vi "Acquire Data.vi"(8 "error in (no error)":errorcluster caption="entrée d'erreur (pas d'erreur)", 11 "Maestro Acq en entrée":refnum<class "Maestro Acq.lvclass">) -> (0 "error out":errorcluster caption="sortie d'erreur", 3 "Maestro Acq en sortie":refnum<class "Maestro Acq.lvclass">)   [LabVIEW 2021, in "Maestro Acq.lvclass"]
uses:
  Maestro Acq.lvclass
  Maestro Acq.lvclass/Maestro Acq.ctl
  4792ea48-66b7-418b-978d-52d7629da4b6.vi
panel:
  out "tableau 2":string[](array[string])
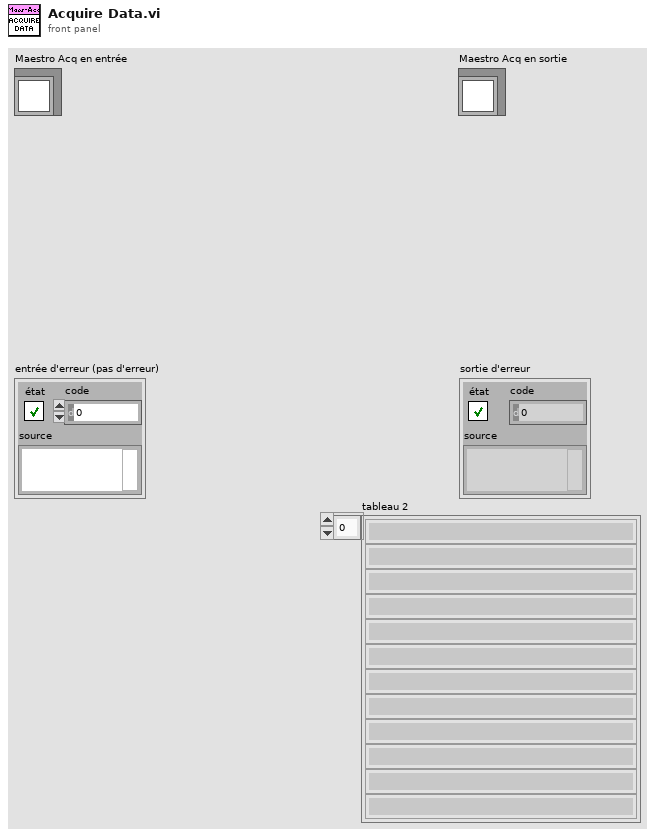
[diagram p1: front panel]
types:
  T1 = enum16{"Standard", "Buffered", "CRLF", "Immediate"}
  T2 = cluster{"Tps(s)":dbl[], "Puiss.":dbl, "Waveform":waveform(dbl)[]}
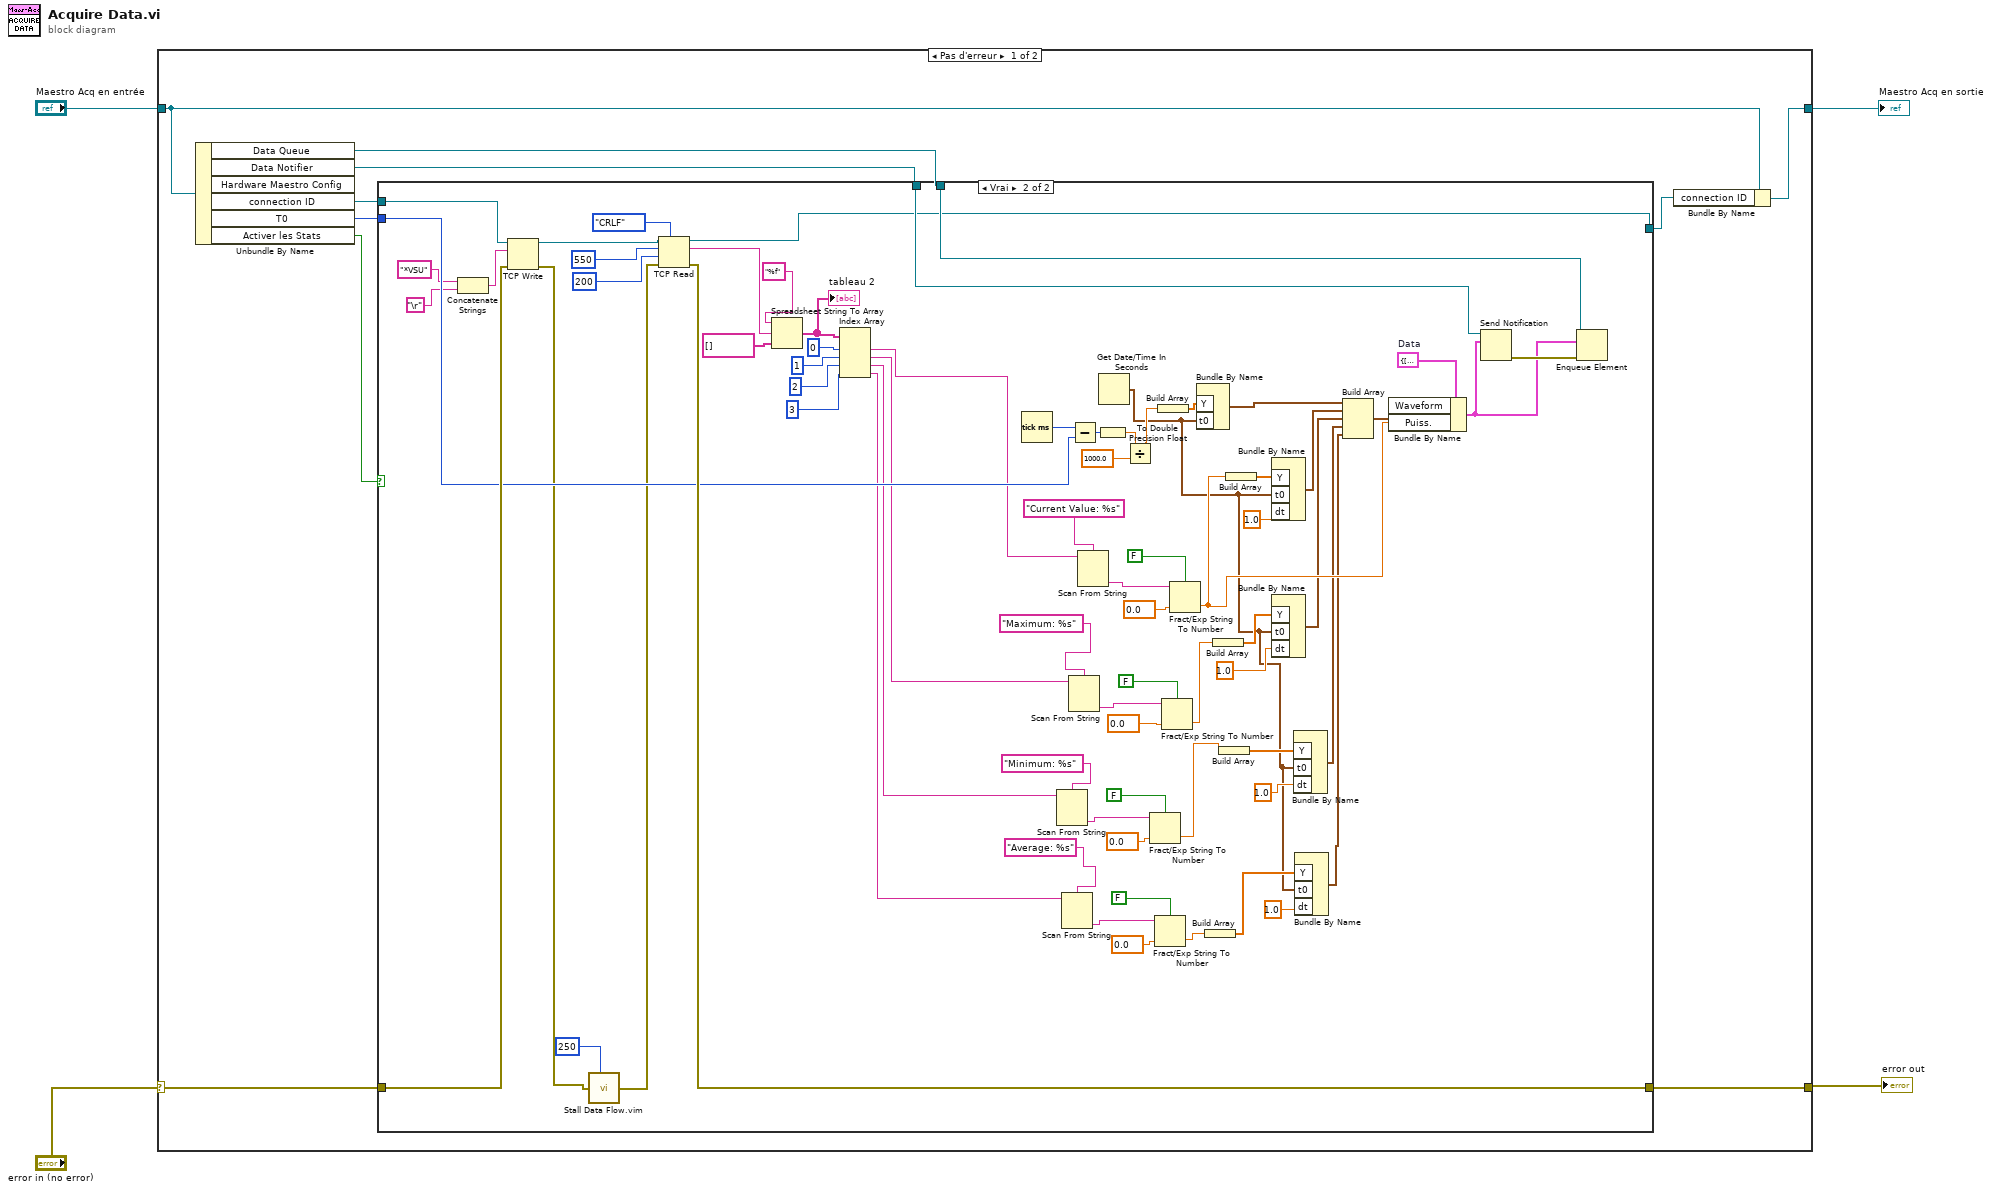
[diagram p0: block diagram]
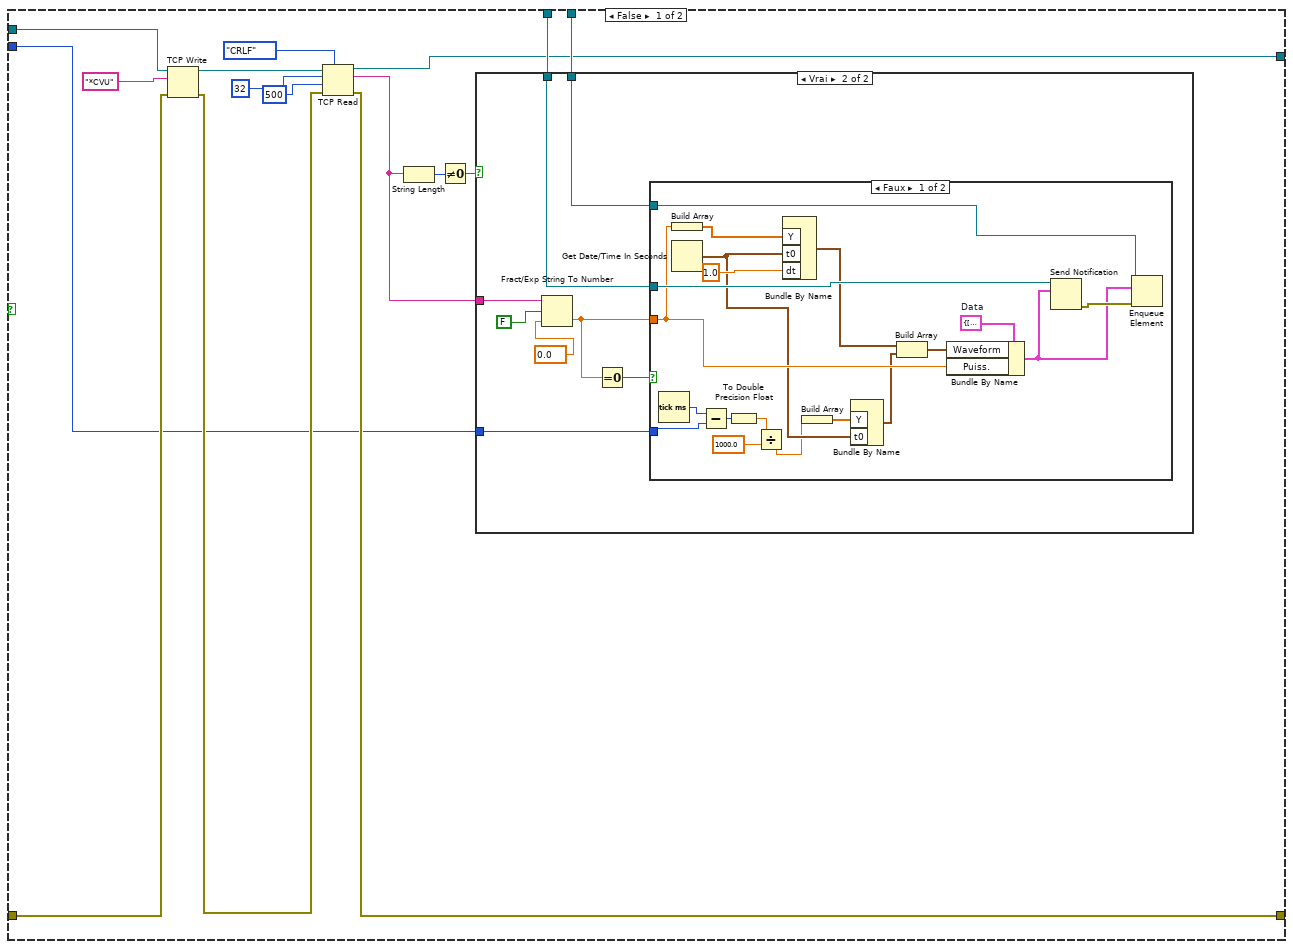
[diagram p2: hidden frame]
diagram:
  n1 = case shown="Pas d'erreur" "error in (no error)" {
    selector: "error in (no error)" -> [w8 w132]
    tunnel: [w12 w132] -> w3
    tunnel: [w14 w131] -> w1
    tunnel: "Maestro Acq en entrée" -> [w13 w131]
    frame No Error {
      n2 = Unbundle By Name(w13) -> ("Data Queue"=w10:refnum<queue>, "Data Notifier"=w11:refnum<notifier>, "connection ID"=w9:refnum<k5>, "T0"=w6:u32, "Activer les Stats"=w5:bool)  [unwired: 1 out]
      n3 = case shown="Vrai" w5 {
        tunnel: [w30 w130] -> w12
        tunnel: w11 -> [w29 w129]
        tunnel: w10 -> [w28 w128]
        tunnel: w9 -> [w27 w127]
        tunnel: w8 -> [w26 w126]
        tunnel: [w22 w122] -> w7
        tunnel: w6 -> [w15 w120]
        frame False {
          n4 = TCP Write(connection ID=w27, data in="*CVU" ("Command"), error in (no error)=w26) -> (connection ID out=w17:refnum<k5>, error out=w16:errorcluster)  [unwired: 1 in, 1 out]
          n5 = TCP Read(connection ID=w17, bytes to read=32, error in (no error)=w16, 7:T1."CRLF" ("mode (standard)"), 9:500 ("timeout ms (25000)")) -> (connection ID out=w22:refnum<k5>, data out=w19:string, error out=w30:errorcluster)
          n6 = String Length(string=w19) -> (length=w21:i32)
          n7 = Not Equal To 0?(x=w21) -> (x != 0?=w20:bool)
          n8 = case shown="Vrai" w20 {
            tunnel: w19 -> [_ w37]
            tunnel: w29 -> [_ w35]
            tunnel: w28 -> [_ w34]
            tunnel: w15 -> [_ w31]
            frame False {
            }
            frame True {
              n9 = Fract/Exp String To Number(use system decimal point (T)=FALSE ("utiliser le séparateur décimal du système (V)"), string=w37, default (0 dbl)=0.0 ("valeur par défaut (0 DBL)")) -> (number=w36:dbl)  [unwired: 1 in, 1 out]
              n10 = Equal To 0?(x=w36) -> (x = 0?=w38:bool)
              n11 = case shown="Faux" w38 {
                tunnel: w36 -> [w49 _]
                tunnel: w35 -> [w57 _]
                tunnel: w34 -> [w56 _]
                tunnel: w31 -> [w46 _]
                frame False {
                  w51 = T2 {"Tps(s)"=[], "Puiss."=0.0, "Waveform"=[]}  # Data
                  n12 = Tick Count (ms)() -> (millisecond timer value=w47:u32)
                  n13 = Build Array(w49) -> (w54:dbl[])
                  n14 = Get Date/Time In Seconds() -> (seconds since 1Jan1904=w44:timestamp)
                  n15 = Subtract(x=w47, y=w46) -> (x-y=w45:u32)
                  n16 = To Double Precision Float(number=w45) -> (double precision float=w41:dbl)
                  n17 = Divide(x=w41, y=1000.0) -> (x/y=w39:dbl)
                  n18 = Bundle By Name("Y"=w54, "t0"=w44, "dt"=1.0) -> (w52:waveform(dbl))  [unwired: 1 in]
                  n19 = Build Array(w39) -> (w42:dbl[])
                  n20 = Bundle By Name("Y"=w42, "t0"=w44) -> (w43:waveform(dbl))  [unwired: 1 in]
                  n21 = Build Array(w52, w43) -> (w50:waveform(dbl)[])
                  n22 = Bundle By Name(cluster=w51, "Waveform"=w50, "Puiss."=w49) -> (w48:T2)
                  n23 = Send Notification(notification=w48, notifier=w57) -> (error out=w55:errorcluster)  [unwired: 1 in, 1 out]
                  n24 = Enqueue Element(queue=w56, element=w48, error in (no error)=w55) -> ()  [unwired: 1 in, 3 out]
                }
                frame True {
                }
              }
            }
          }
        }
        frame True {
          w103 = T2 {"Tps(s)"=[], "Puiss."=0.0, "Waveform"=[]}  # Data
          n25 = Concatenate Strings("*VSU" ("Command"), "\r") -> (w59:string)
          n26 = TCP Write(connection ID=w127, data in=w59, error in (no error)=w126) -> (connection ID out=w121:refnum<k5>, error out=w107:errorcluster)  [unwired: 1 in, 1 out]
          n27 = call "Stall Data Flow.vim"("value in"=w107, "milliseconds to wait"=u32 250) -> ("value out"=w106:errorcluster)  [unwired: 1 out]
          n28 = TCP Read(connection ID=w121, bytes to read=550, error in (no error)=w106, 7:T1."CRLF" ("mode (standard)"), 9:200 ("timeout ms (25000)")) -> (connection ID out=w122:refnum<k5>, data out=w115:string, error out=w130:errorcluster)
          n29 = Spreadsheet String To Array(format string="%f", spreadsheet string=w115, array type (2D Dbl)=string[] [] ("Array")) -> (array=w116:string[])  [unwired: 1 in]
          "tableau 2" <- w116
          n30 = Index Array(array=w116, index #1=0 ("indice"), index #2=1 ("indice"), index #3=2 ("indice"), index #4=3 ("indice")) -> (element #1=w114:string, element #2=w110:string, element #3=w109:string, element #4=w108:string)
          n31 = Tick Count (ms)() -> (millisecond timer value=w101:u32)
          n32 = Scan From String(format string="Minimum: %s", input string=w109) -> (output 1=w74:string)  [unwired: 3 in, 3 out]
          n33 = Scan From String(format string="Average: %s", input string=w108) -> (output 1=w69:string)  [unwired: 3 in, 3 out]
          n34 = Scan From String(format string="Maximum: %s", input string=w110) -> (output 1=w85:string)  [unwired: 3 in, 3 out]
          n35 = Subtract(x=w101, y=w120) -> (x-y=w100:u32)
          n36 = Scan From String(format string="Current Value: %s" ("chaîne de format"), input string=w114) -> (output 1=w94:string)  [unwired: 3 in, 3 out]
          n37 = To Double Precision Float(number=w100) -> (double precision float=w98:dbl)
          n38 = Get Date/Time In Seconds() -> (seconds since 1Jan1904=w62:timestamp)
          n39 = Divide(x=w98, y=1000.0) -> (x/y=w96:dbl)
          n40 = Fract/Exp String To Number(use system decimal point (T)=FALSE ("utiliser le séparateur décimal du système (V)"), string=w74, default (0 dbl)=0.0 ("valeur par défaut (0 DBL)")) -> (number=w73:dbl)  [unwired: 1 in, 1 out]
          n41 = Fract/Exp String To Number(use system decimal point (T)=FALSE ("utiliser le séparateur décimal du système (V)"), string=w69, default (0 dbl)=0.0 ("valeur par défaut (0 DBL)")) -> (number=w65:dbl)  [unwired: 1 in, 1 out]
          n42 = Build Array(w96) -> (w99:dbl[])
          n43 = Fract/Exp String To Number(use system decimal point (T)=FALSE ("utiliser le séparateur décimal du système (V)"), string=w85, default (0 dbl)=0.0 ("valeur par défaut (0 DBL)")) -> (number=w81:dbl)  [unwired: 1 in, 1 out]
          n44 = Fract/Exp String To Number(use system decimal point (T)=FALSE ("utiliser le séparateur décimal du système (V)"), string=w94, default (0 dbl)=0.0 ("valeur par défaut (0 DBL)")) -> (number=w88:dbl)  [unwired: 1 in, 1 out]
          n45 = Bundle By Name("Y"=w99, "t0"=w62) -> (w95:waveform(dbl))  [unwired: 1 in]
          n46 = Build Array(w65) -> (w64:dbl[])
          n47 = Build Array(w81) -> (w80:dbl[])
          n48 = Build Array(w73) -> (w72:dbl[])
          n49 = Build Array(w88) -> (w90:dbl[])
          n50 = Bundle By Name("Y"=w90, "t0"=w62, "dt"=1.0) -> (w87:waveform(dbl))  [unwired: 1 in]
          n51 = Bundle By Name("Y"=w80, "t0"=w62, "dt"=1.0) -> (w78:waveform(dbl))  [unwired: 1 in]
          n52 = Bundle By Name("Y"=w72, "t0"=w62, "dt"=1.0) -> (w70:waveform(dbl))  [unwired: 1 in]
          n53 = Bundle By Name("Y"=w64, "t0"=w62, "dt"=1.0) -> (w61:waveform(dbl))  [unwired: 1 in]
          n54 = Build Array(w95, w87, w78, w70, w61) -> (w86:waveform(dbl)[])
          n55 = Bundle By Name(cluster=w103, "Waveform"=w86, "Puiss."=w88) -> (w102:T2)
          n56 = Send Notification(notification=w102, notifier=w129) -> (error out=w104:errorcluster)  [unwired: 1 in, 1 out]
          n57 = Enqueue Element(queue=w128, element=w102, error in (no error)=w104) -> ()  [unwired: 1 in, 3 out]
        }
      }
      n58 = Bundle By Name(cluster=w13, "connection ID"=w7) -> (w14:refnum<class "Maestro Acq.lvclass">)
    }
    frame Error {
    }
  }
  "error out" <- w3
  "Maestro Acq en sortie" <- w1
